vi "Compute DistanceToTarget (Modified).vi"(8 "Y Image Resolution":i32, 9 "X Image Resolution":i32, 10 "Vertical Strip":T1, 11 "Camera Type":enum16{"206", "1011", "1013"}(ring)) -> (0 "Distance to Strip (ft)":dbl, 2 "Target Center (-1 to 1)":cluster{"X":dbl, "Y":dbl}, 3 "Distance to Goal Wall (ft)":dbl)   [LabVIEW 2013]
doc: "Using the camera lens information and the real world size of the target, use trig and ratios to determine the distance to the target. Also returns the location relative to the image center in a (-1 , 1) coordinate system that may be useful for steering the robot."
panel:
  in  "Camera view angles":dbl[](array[numeric])=[41.7, 37.4, 49.0]
  # "Axis 206\nAxis M1011\nAxis M1013"
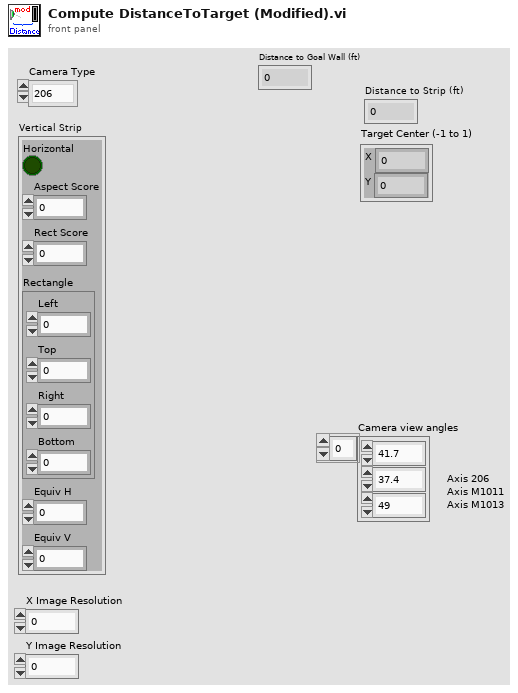
[diagram p1: front panel]
types:
  T1 = cluster{"Horizontal":bool, "Aspect Score":dbl, "Rect Score":dbl, "Rectangle":cluster{"Left":dbl, "Top":dbl, "Right":dbl, "Bottom":dbl}, "Equiv H":dbl, "Equiv V":dbl}
  T2 = cluster{"X Image Resolution":i32, "Y Image Resolution":i32}
  T3 = cluster{"X Image Resolution":dbl, "Y Image Resolution":dbl}
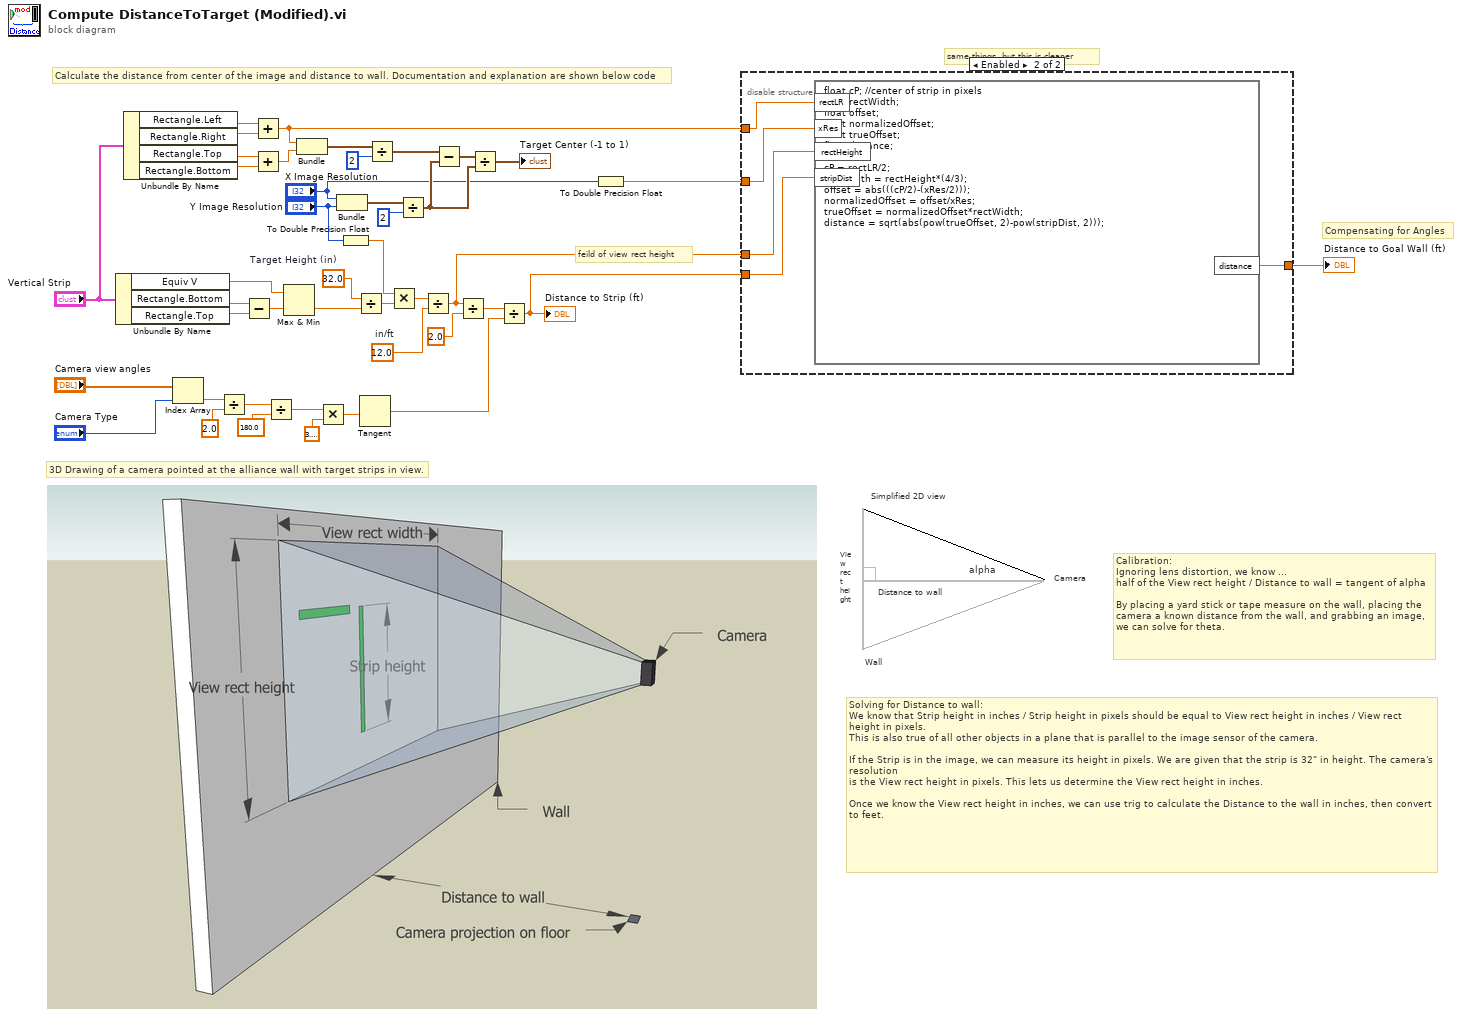
[diagram p0: block diagram]
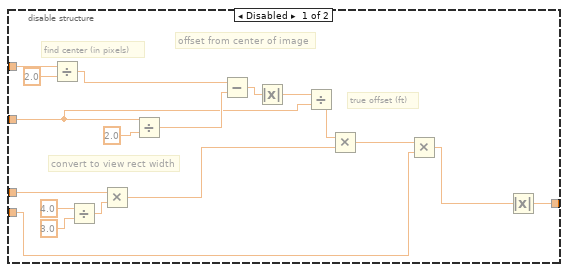
[diagram p2: hidden frame]
diagram:
  w12 = 12.0  # in/ft
  w17 = 32.0  # Target Height (in)
  # "Compensating for Angles"
  # "same things, but this is cleaner"
  # "feild of view rect height"
  # "Wall"
  # "Camera"
  # "Simplified 2D view"
  # "Solving for Distance to wall:\nWe know that Strip height in inches / Strip height in pixels should be equal to View rect height in inches / View rect height in pixels.\nThis is also true of all other objects in a plane that is parallel to the image sensor of the camera.\n\nIf the Strip is in the image, we can measure its height in pixels. We are given that the strip is 32\" in height. The camera's resolution\nis the View rect height in pixels. This lets us determine the View rect height in inches.\n\nOnce we know the View rect height in inches, we can use trig to calculate the Distance to the wall in inches, then convert to feet."
  # "3D Drawing of a camera pointed at the alliance wall with target strips in view."
  # "Distance to wall"
  # "View rect height"
  # "alpha"
  # "Calibration:\nIgnoring lens distortion, we know ...\nhalf of the View rect height / Distance to wall = tangent of alpha\n\nBy placing a yard stick or tape measure on the wall, placing the\ncamera a known distance from the wall, and grabbing an image,\nwe can solve for theta."
  # "Calculate the distance from center of the image and distance to wall. Documentation and explanation are shown below code"
  n1 = Unbundle By Name("Vertical Strip") -> ("Equiv V"=w19:dbl, "Rectangle.Bottom"=w34:dbl, "Rectangle.Top"=w33:dbl)
  n2 = Unbundle By Name("Vertical Strip") -> ("Rectangle.Left"=w28:dbl, "Rectangle.Right"=w29:dbl, "Rectangle.Top"=w31:dbl, "Rectangle.Bottom"=w30:dbl)
  n3 = Index Array(array="Camera view angles", index="Camera Type") -> (element=w40:dbl)
  n4 = Divide(x=w40, y=2.0) -> (x/y=w37:dbl)
  n5 = Subtract(x=w34, y=w33) -> (x-y=w18:dbl)
  n6 = Add(x=w28, y=w29) -> (x+y=w4:dbl)
  n7 = Add(x=w31, y=w30) -> (x+y=w26:dbl)
  n8 = Divide(x=w37, y=180.0) -> (x/y=w36:dbl)
  n9 = Max & Min(x=w19, y=w18) -> (min(x,y)=w16:dbl)  [unwired: 1 out]
  n10 = Bundle(w4, w26) -> (w23:cluster{dbl, dbl})  [unwired: 1 in]
  n11 = Multiply(x=w36, y=3.141592653589793) -> (x*y=w38:dbl)
  n12 = Bundle("X Image Resolution"="X Image Resolution", "Y Image Resolution"="Y Image Resolution") -> (w25:T2)  [unwired: 1 in]
  n13 = To Double Precision Float(number="Y Image Resolution") -> (double precision float=w1:dbl)
  n14 = Divide(x=w17, y=w16) -> (x/y=w15:dbl)
  n15 = Tangent(1:w38) -> (0:w9:dbl)
  n16 = Divide(x=w23, y=2) -> (x/y=w8:cluster{dbl, dbl})
  n17 = Multiply(x=w1, y=w15) -> (x*y=w13:dbl)
  n18 = Divide(x=w25, y=2) -> (x/y=w21:T3)
  n19 = Divide(x=w13, y=w12) -> (x/y=w5:dbl)
  n20 = Subtract(x=w8, y=w21) -> (x-y=w22:cluster{dbl, dbl})
  n21 = Divide(x=w5, y=2.0) -> (x/y=w10:dbl)
  n22 = Divide(x=w22, y=w21) -> (x/y=→"Target Center (-1 to 1)":cluster{dbl, dbl})
  n23 = Divide(x=w10, y=w9) -> (x/y=w2:dbl)
  "Distance to Strip (ft)" <- w2
  n24 = To Double Precision Float(number="X Image Resolution") -> (double precision float=w3:dbl)
  n25 = disable-structure shown="Enabled" {
    disable-tunnel: [w44 w63] -> w6
    disable-tunnel: w5 -> [w49 w65]
    disable-tunnel: w4 -> [w48 w66]
    disable-tunnel: w3 -> [w47 w64]
    disable-tunnel: w2 -> [w45 w62]
    frame Disabled {
      # "true offset (ft)"
      # "offset from center of image"
      # "find center (in pixels)"
      # "convert to view rect width"
      n26 = Divide(x=w48, y=2.0) -> (x/y=w50:dbl)
      n27 = Divide(x=4.0, y=3.0) -> (x/y=w61:dbl)
      n28 = Multiply(x=w49, y=w61) -> (x*y=w57:dbl)
      n29 = Divide(x=w47, y=2.0) -> (x/y=w55:dbl)
      n30 = Subtract(x=w50, y=w55) -> (x-y=w54:dbl)
      n31 = Absolute Value(x=w54) -> (abs(x)=w53:dbl)
      n32 = Divide(x=w53, y=w47) -> (x/y=w51:dbl)
      n33 = Multiply(x=w51, y=w57) -> (x*y=w52:dbl)
      n34 = Multiply(x=w52, y=w45) -> (x*y=w46:dbl)
      n35 = Absolute Value(x=w46) -> (abs(x)=w44:dbl)
    }
    frame Enabled {
      n36 = formula code="float cP; //center of strip in pixels\nfloat rectWidth;\nfloat offset;\nfloat normalizedOffset;\nfloat trueOffset;\nfloat distance;\n\ncP = rectLR/2;\nrectWidth = rectHeight*(4/3);\noffset = abs(((cP/2)-(xRes/2)));\nnormalizedOffset = offset/xRes;\ntrueOffset = normalizedOffset*rectWidth;\ndistance = sqrt(abs(pow(trueOffset, 2)-pow(stripDist, 2)));"("rectLR"=w66, "rectHeight"=w65, "xRes"=w64, "stripDist"=w62) -> ("distance"=w63:dbl)
    }
  }
  "Distance to Goal Wall (ft)" <- w6
